vi "Read Method Results.vi"(11 "Test Case Result In":T5) -> (2 "Method Results":map{string, T1}(c390), 3 "Test Case Result Out":T5)   [LabVIEW 2020, in "Test Case Result.lvlib"]
uses:
  Test Case Result.lvlib
  Test Case Result.ctl
  Method Result/Method Result.ctl
  Rewrite Project/Result/Status.ctl
  Assertion Result/Assertion Result.ctl
  Assertion Result/Public/TypeDefs/Assertion Type.ctl
  Assertion Result/Assertion Result.lvlib
  Method Result/Method Result.lvlib
  Rewrite Project/Result/Result.lvlib
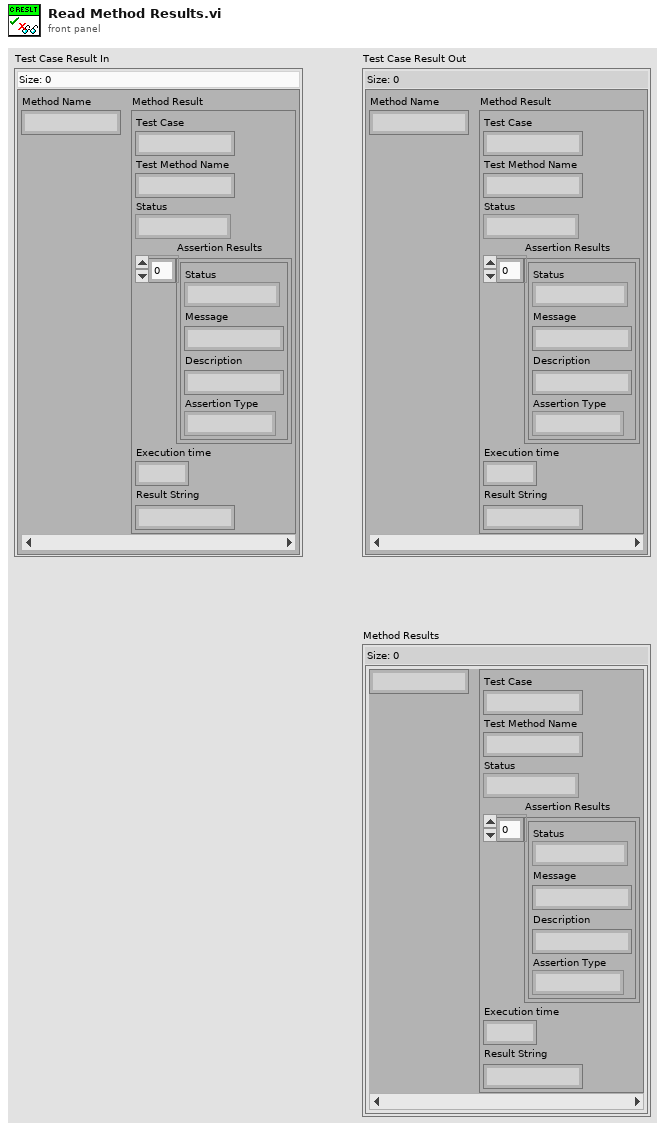
[diagram p1: front panel]
types:
  T1 = typedef "Method Result.lvlib/Method Result.ctl" = cluster{"Test Case":string, "Test Method Name":string, "Status":T2, "Assertion Results":T3[], "Execution time":dbl, "Result String":string}
  T2 = typedef "Result.lvlib/Status.ctl" = enum16{"Pass", "Fail", "Error", "Skipped", "Setup Error", "Broken", "Teardown Error"}
  T3 = typedef "Assertion Result.lvlib/Assertion Result.ctl" = cluster{"Status":T2, "Message":string, "Description":string, "Assertion Type":T4}
  T4 = typedef "Result.lvlib/Assertion Type.ctl" = enum16{"None", "Pass", "Fail", "Skip", "Pass if Equal", "Fail if Equal", "Pass if Error", "Fail if Error", "Pass if", "Fail if"}
  T5 = typedef "Test Case Result.lvlib/Test Case Result.ctl" = map{string, T1}
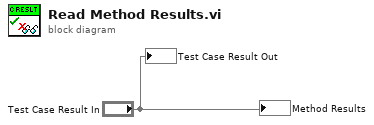
[diagram p0: block diagram]
diagram:
  "Test Case Result Out" <- "Test Case Result In"
  "Method Results" <- "Test Case Result In"
